vi "dispatcher core.vi"(7 "action":enum16{"init", "read", "write"}(ring), 8 "error in (no error)":errorcluster, 9 "control value (in)":string, 10 "control name":string, 11 "vi path":path=path "C:/LabVIEW/LV Py/demo target.vi") -> (0 "error out":errorcluster, 1 "control value (out)":string)   [LabVIEW 2025]
doc: "Use the <b>init</b> action to find all the controls on the VI [vi path] under control.\n\nUse the <b>read</b> action to read a value [control value (out)] from a given control ([control name]). This method can be used for reading a single element from an array or a specific individual value from a cluster.\nCommon scalar values, entire arrays and clusters, can be read by Python directly.\n\nUse the <b>write</b> action to write a value [control value (in)] to a given control ([control name]).\nThis method can be used if changing the value of a control should trigger event. This method can also be used for writing a single element in an array or a specific individual value in a cluster. \nCommon scalar values, entire arrays and clusters, can be written by Python directly."
uses:
  dispatcher.llb/gc - controlspecs.ctl
  <vilib>/Utility/Data Type/NI_Data Type.lvlib
panel:
  in  "Enum":enum16{""}(ring)
  out "control specs":T1[](array[typedef])
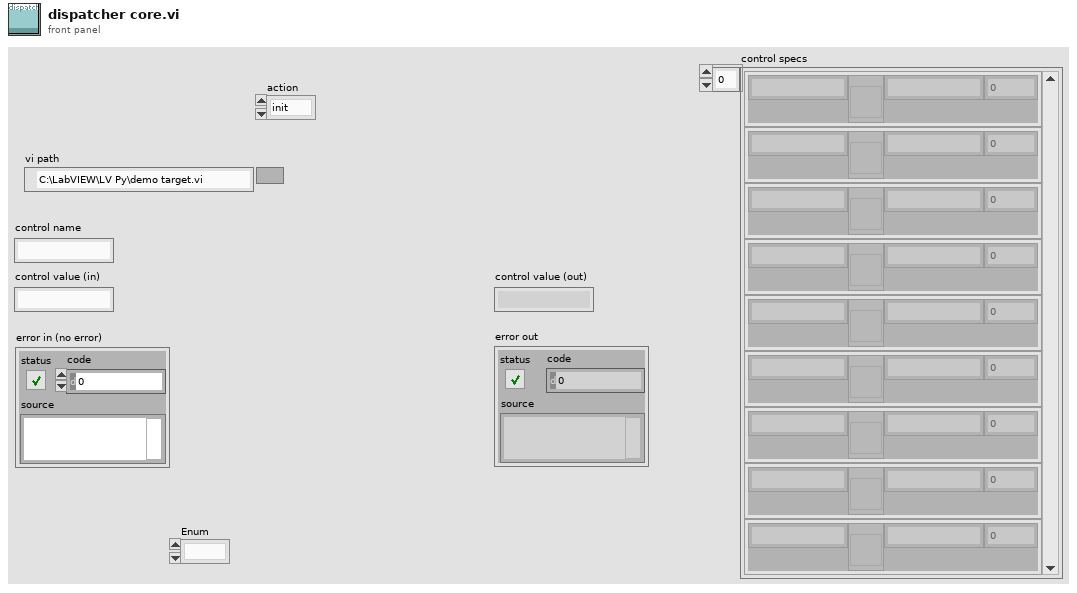
[diagram p1: front panel]
types:
  T1 = typedef "gc - controlspecs.ctl" = cluster{"name":string, "reference":refnum<vi>, "type":string, "idx":i32}
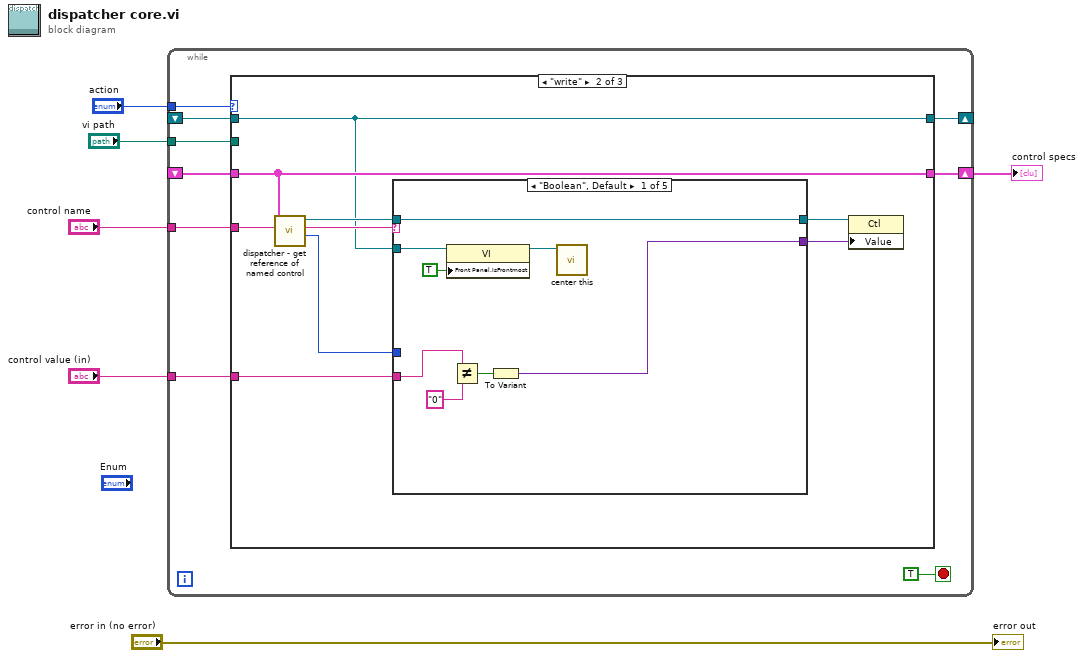
[diagram p0: block diagram]
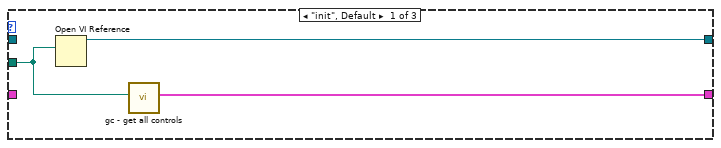
[diagram p2: hidden frame]
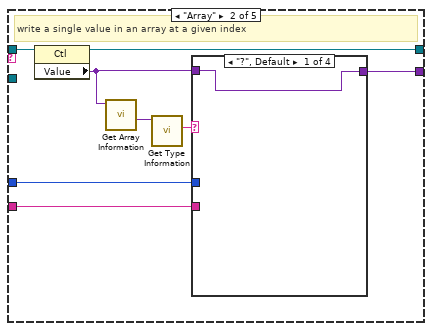
[diagram p3: hidden frame]
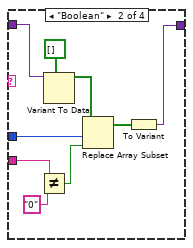
[diagram p4: hidden frame]
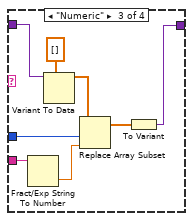
[diagram p5: hidden frame]
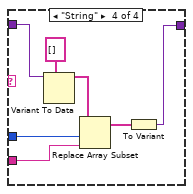
[diagram p6: hidden frame]
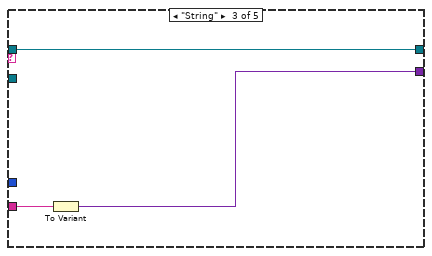
[diagram p7: hidden frame]
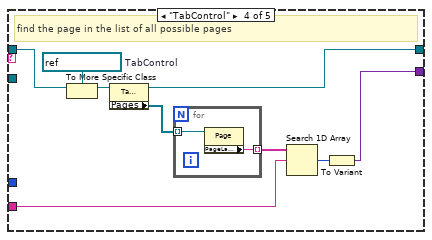
[diagram p8: hidden frame]
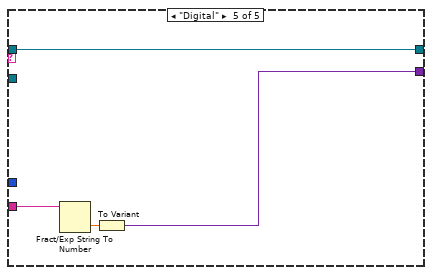
[diagram p9: hidden frame]
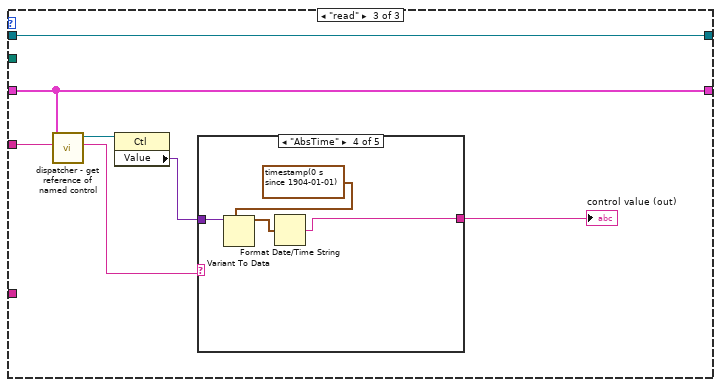
[diagram p10: hidden frame]
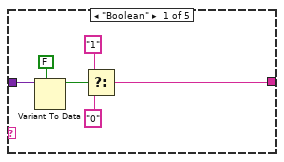
[diagram p11: hidden frame]
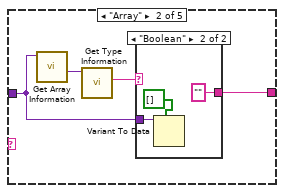
[diagram p12: hidden frame]
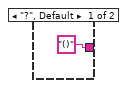
[diagram p13: hidden frame]
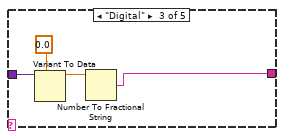
[diagram p14: hidden frame]
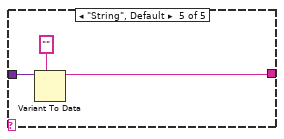
[diagram p15: hidden frame]
diagram:
  n1 = while {
    tunnel: "action" -> [w14]
    tunnel: "vi path" -> [w13]
    tunnel: "control name" -> [w12]
    shift-right: [w11] -> w1
    shift-left: _ -> [w10]
    tunnel: "control value (in)" -> [w9]
    shift-right: [w8] -> _
    shift-left: _ -> [w7]
    stop <- TRUE stop-if-true
    n2 = case shown="\"write\"" w14 {
      tunnel: w13 -> [w17 _ _]
      tunnel: w12 -> [_ w27 w93]
      tunnel: [w18 w26 w92] -> w11
      tunnel: w10 -> [_ w26 w92]
      tunnel: w9 -> [_ w25 _]
      tunnel: [w16 w19 w87] -> w8
      tunnel: w7 -> [_ w19 w87]
      frame "init", Default {
        n3 = Open VI Reference(vi path=w17) -> (vi reference=w16:refnum<vi>)  [unwired: 5 in, 1 out]
        n4 = call "gc - get all controls.vi"("vi path"=w17) -> ("control specs"=w18:T1[])  [unwired: 7 in, 3 out]
      }
      frame "write" {
        n5 = call "dispatcher - get reference of named control.vi"("named control"=w27, "control specs"=w26) -> ("idx"=w22:i32, "type"=w23:string, "reference"=w21:refnum<vi>)  [unwired: 5 in, 1 out]
        n6 = case shown="\"Boolean\", Default" w23 {
          tunnel: w25 -> [w35 w38 w70 w73 w86]
          tunnel: [w33 w36 w71 w80 w84] -> w24
          tunnel: w22 -> [_ w37 _ _ _]
          tunnel: w21 -> [w31 w43 w69 w78 w83]
          tunnel: [w31 w41 w69 w79 w83] -> w20
          tunnel: w19 -> [w29 _ _ _ _]
          frame "Boolean", Default {
            n7 = property class="VI"(reference=w29, "Front Panel.IsFrontmost"=TRUE ("Front Panel Window:Is Frontmost")) -> (reference out=w28:refnum<vi>)  [unwired: 1 in, 1 out]
            n8 = Not Equal?(x=w35, y="0") -> (x != y?=w32:bool)
            n9 = To Variant(anything=w32) -> (Variant=w33:variant)
            n10 = call "center this.vi"("vi reference"=w28) -> ()  [unwired: 11 in]
          }
          frame "Array" {
            # "write a single value in an array at a given index"
            n11 = property class="Ctl"(reference=w43) -> (reference out=w41:refnum<vi>, "Value"=w39:variant)  [unwired: 1 in, 1 out]
            n12 = call <vilib>:"Get Array Information.vi"("variant"=w39) -> ("array element data type"=w42:variant)  [unwired: 7 in, 3 out]
            n13 = call <vilib>:"Get Type Information.vi"("variant"=w42) -> ("name"=w40:string)  [unwired: 6 in, 4 out]
            n14 = case shown="\"?\", Default" w40 {
              tunnel: w39 -> [w44 w53 w61 w68]
              tunnel: w38 -> [_ w50 w55 w62]
              tunnel: w37 -> [_ w48 w58 w65]
              tunnel: [w44 w45 w56 w63] -> w36
              frame "?", Default {
              }
              frame "Boolean" {
                n15 = Not Equal?(x=w50, y="0") -> (x != y?=w47:bool)
                n16 = Variant To Data(type=bool[] [], Variant=w53) -> (data=w49:bool[])  [unwired: 1 in, 1 out]
                n17 = Replace Array Subset(array=w49, new element=w47, index=w48) -> (w46:bool[])
                n18 = To Variant(anything=w46) -> (Variant=w45:variant)
              }
              frame "Numeric" {
                n19 = Fract/Exp String To Number(string=w55) -> (number=w54:dbl)  [unwired: 3 in, 1 out]
                n20 = Variant To Data(type=dbl[] [], Variant=w61) -> (data=w59:dbl[])  [unwired: 1 in, 1 out]
                n21 = Replace Array Subset(array=w59, new element=w54, index=w58) -> (w57:dbl[])
                n22 = To Variant(anything=w57) -> (Variant=w56:variant)
              }
              frame "String" {
                n23 = Variant To Data(type=string[] [], Variant=w68) -> (data=w66:string[])  [unwired: 1 in, 1 out]
                n24 = Replace Array Subset(array=w66, new element=w62, index=w65) -> (w64:string[])
                n25 = To Variant(anything=w64) -> (Variant=w63:variant)
              }
            }
          }
          frame "String" {
            n26 = To Variant(anything=w70) -> (Variant=w71:variant)
          }
          frame "TabControl" {
            w76 = refnum<vi> refnum  # TabControl
            # "find the page in the list of all possible pages"
            n27 = To More Specific Class(target class=w76, reference=w78) -> (specific class reference=w77:refnum<vi>)  [unwired: 1 in, 1 out]
            n28 = property class="TabCtl"(reference=w77) -> (reference out=w79:refnum<vi>, "Pages"=w75:refnum<vi>[])  [unwired: 1 in, 1 out]
            n29 = for {
              tunnel: w75 -> [w82] mode=indexing
              tunnel: [w81] -> w74 mode=indexing
              n30 = property class="Page"(reference=w82) -> ("PageLabel"=w81:string)  [unwired: 1 in, 2 out]
            }
            n31 = Search 1D Array(1D array=w74, element=w73) -> (index of element=w72:i32)  [unwired: 1 in]
            n32 = To Variant(anything=w72) -> (Variant=w80:variant)
          }
          frame "Digital" {
            n33 = Fract/Exp String To Number(string=w86) -> (number=w85:dbl)  [unwired: 3 in, 1 out]
            n34 = To Variant(anything=w85) -> (Variant=w84:variant)
          }
        }
        n35 = property class="Ctl"(reference=w20, "Value"=w24) -> ()  [unwired: 1 in, 2 out]
      }
      frame "read" {
        n36 = call "dispatcher - get reference of named control.vi"("named control"=w93, "control specs"=w92) -> ("type"=w90:string, "reference"=w91:refnum<vi>)  [unwired: 5 in, 2 out]
        n37 = property class="Ctl"(reference=w91) -> ("Value"=w89:variant)  [unwired: 1 in, 2 out]
        n38 = case shown="\"AbsTime\"" w90 {
          tunnel: w89 -> [w99 w103 w111 w115 w118]
          tunnel: [w94 w100 w108 w114 w116] -> w88
          frame "Boolean" {
            n39 = Variant To Data(type=FALSE, Variant=w99) -> (data=w96:bool)  [unwired: 1 in, 1 out]
            n40 = Select(t="1", s=w96, f="0") -> (s? t:f=w94:string)
          }
          frame "Array" {
            n41 = call <vilib>:"Get Array Information.vi"("variant"=w103) -> ("array element data type"=w102:variant)  [unwired: 7 in, 3 out]
            n42 = call <vilib>:"Get Type Information.vi"("variant"=w102) -> ("name"=w101:string)  [unwired: 6 in, 4 out]
            n43 = case shown="\"Boolean\"" w101 {
              tunnel: w103 -> [_ w107]
              tunnel: ["()" ""] -> w100
              frame "?", Default {
              }
              frame "Boolean" {
                n44 = Variant To Data(type=bool[] [], Variant=w107) -> ()  [unwired: 1 in, 2 out]
              }
            }
          }
          frame "Digital" {
            n45 = Variant To Data(type=0.0, Variant=w111) -> (data=w109:dbl)  [unwired: 1 in, 1 out]
            n46 = Number To Fractional String(number=w109) -> (F-format string=w108:string)  [unwired: 3 in]
          }
          frame "AbsTime" {
            n47 = Variant To Data(type=timestamp(0 s since 1904-01-01), Variant=w115) -> (data=w112:timestamp)  [unwired: 1 in, 1 out]
            n48 = Format Date/Time String(seconds (now)=w112) -> (date/time string=w114:string)  [unwired: 2 in]
          }
          frame "String", Default {
            n49 = Variant To Data(type="", Variant=w118) -> (data=w116:string)  [unwired: 1 in, 1 out]
          }
        }
        "control value (out)" <- w88
      }
    }
  }
  "control specs" <- w1
  "error out" <- "error in (no error)"
